vi "Find SLSC Switch Custom Device by Name.vi"(8 "error in (no error)":errorcluster, 10 "Name":string, 11 "Target in":refnum<k24>) -> (0 "error out":errorcluster, 2 "SLSC Switch Custom Device Ref":T1 format="%.0x", 3 "Target out":refnum<k24>)   [LabVIEW 2017, in "SLSC Switch Scripting.lvlib"]
uses:
  SLSC Switch Scripting.lvlib
  NationalInstruments.VeriStand.SystemDefinitionAPI
  <vilib>/NI Veristand/Custom Device API/Custom Device Item Ref.ctl
  Shared/Constants.vi
  Shared/SLSC Switch Shared.lvlib
  <vilib>/NI Veristand/Custom Device API/Custom Device API.lvlib
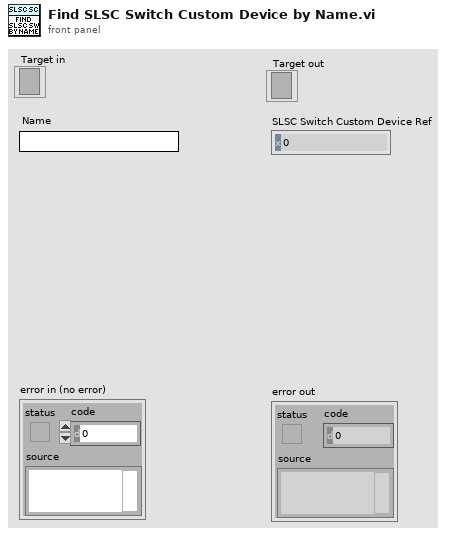
[diagram p1: front panel]
types:
  T1 = typedef "Custom Device API.lvlib/Custom Device Item Ref.ctl" = u64
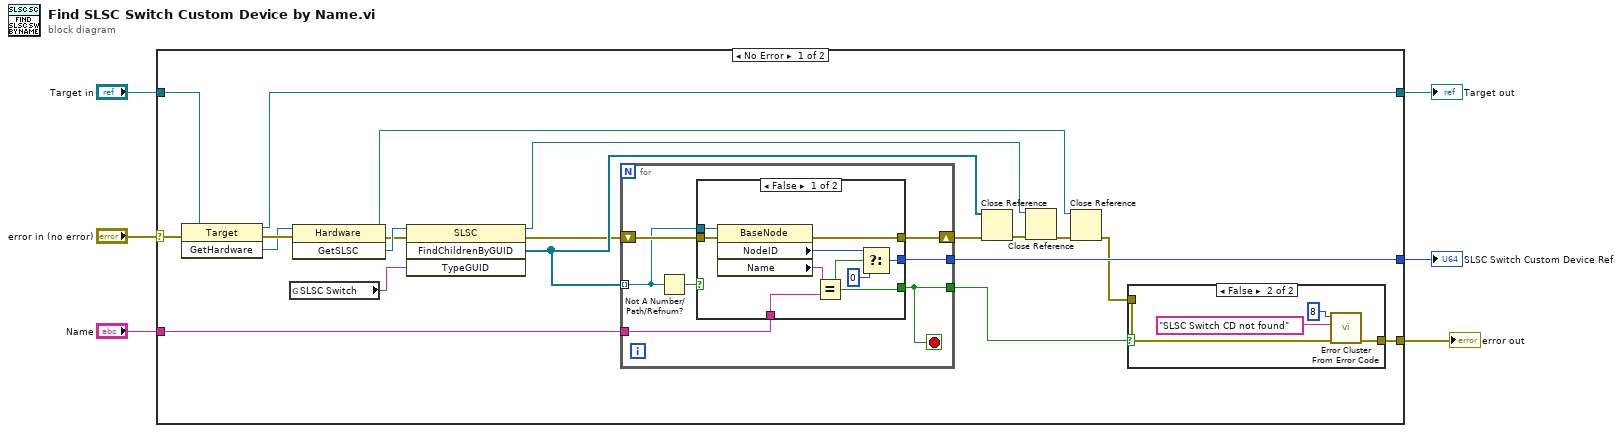
[diagram p0: block diagram]
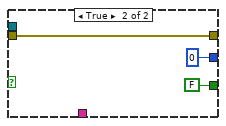
[diagram p3: hidden frame]
diagram:
  n1 = case shown="No Error" "error in (no error)" {
    selector: "error in (no error)" -> [w20 w52]
    tunnel: [w9 w52] -> w6
    tunnel: "Target in" -> [w24 w51]
    tunnel: "Name" -> [w7 _]
    tunnel: [w26 _] -> w2
    tunnel: [w19 w51] -> w1
    frame No Error {
      n2 = invoke class="Target" method="GetHardware"(reference=w24, error in=w20) -> (reference out=w19:refnum<k24>, error out=w23:errorcluster, "GetHardware"=w22:refnum<k24>)  [unwired: 1 in]
      n3 = global read "Constants.vi" "SLSC Switch"() -> (w8:string)
      n4 = invoke class="Hardware" method="GetSLSC"(reference=w22, error in=w23) -> (reference out=w12:refnum<k24>, error out=w17:errorcluster, "GetSLSC"=w21:refnum<k24>)  [unwired: 1 in]
      n5 = invoke class="SLSC" method="FindChildrenByGUID"(reference=w21, error in=w17, "TypeGUID"=w8) -> (reference out=w13:refnum<k24>, error out=w18:errorcluster, "FindChildrenByGUID"=w25:refnum<k24>[])  [unwired: 1 in, 1 out]
      n6 = for {
        tunnel: w25 -> [w36] mode=indexing
        shift-right: [w35] -> w16
        shift-left: w18 -> [w38]
        tunnel: w7 -> [w34]
        tunnel: [w33] -> w26
        tunnel: [w32] -> w10
        stop <- w32 stop-if-true
        n7 = Not A Number/Path/Refnum?(number/path/refnum=w36) -> (NaN/Path/Refnum?=w37:bool)
        n8 = case shown="False" w37 {
          tunnel: w38 -> [w47 w49]
          tunnel: [w39 u64 0 ("f")] -> w33
          tunnel: w36 -> [w46 _]
          tunnel: [w42 FALSE] -> w32
          tunnel: [w43 w49] -> w35
          tunnel: w34 -> [w44 _]
          frame False {
            n9 = property class="BaseNode"(reference=w46, error in=w47) -> (error out=w43:errorcluster, "NodeID"=w41:u64, "Name"=w45:string)  [unwired: 1 out]
            n10 = Equal?(x=w45, y=w44) -> (x = y?=w42:bool)
            n11 = Select(t=w41, s=w42, f=u64 0) -> (s? t:f=w39:u64)
          }
          frame True {
          }
        }
      }
      n12 = Close Reference(reference=w25, error in (no error)=w16) -> (error out=w15:errorcluster)
      n13 = Close Reference(reference=w13, error in (no error)=w15) -> (error out=w14:errorcluster)
      n14 = Close Reference(reference=w12, error in (no error)=w14) -> (error out=w11:errorcluster)
      n15 = case shown="False" w10 {
        tunnel: [w27 w29] -> w9
        tunnel: w11 -> [w27 w28]
        frame True {
        }
        frame False {
          n16 = call <vilib>:"Error Cluster From Error Code.vi"("error in (no error)"=w28, "error message (\"\")"="SLSC Switch CD not found" ("error message (\"\")"), "error code (0)"=8) -> ("error out"=w29:errorcluster)  [unwired: 6 in]
        }
      }
    }
    frame Error {
    }
  }
  "Target out" <- w1
  "error out" <- w6
  "SLSC Switch Custom Device Ref" <- w2
